vi "dummy RPM.vi"() -> ()   [LabVIEW 2018]
uses:
  <vilib>/DAQmx/write.llb/DAQmx Write (Counter Frequency 1Chan 1Samp).vi
  <vilib>/addons/control/pid/NI_PID_pid.lvlib
  <vilib>/DAQmx/configure/timing.llb/DAQmx Timing (Implicit).vi
  <vilib>/addons/control/pid/_prctrl compat.llb/PID (Compatibility).vi
  <vilib>/addons/control/pid/NI_PID__prctrl compat.lvlib
  <vilib>/DAQmx/read.llb/DAQmx Read (Counter DBL 1Chan 1Samp).vi
  <vilib>/addons/control/pid/pid.llb/PID Percentage to EGU (DBL).vi
panel:
  out "error":dbl
  in  "PID parameters":cluster{"Kp":dbl, "Ti":dbl, "Td":dbl}={"Kp"=1.0, "Ti"=0.0, "Td"=0.0} {"Td" format="%.2f"; "Ti" format="%.2f"; "Kp" format="%.2f"}
  out "Process Variable":dbl(knob) scale=0.0..180.0
  in  "Setpoint":dbl(knob) scale=0.0..180.0
  in  "frequency":dbl=1.0 format="%_6g"
  out "Respuesta":cluster{"Setpoint":dbl, "RPM":dbl, dbl}(graph)
  in  "stop":bool
  # "Proportional gain or band (Kc)"
  # "Integral (reset) time (Ti, min)"
  # "Derivative (rate) time (Td, min)"
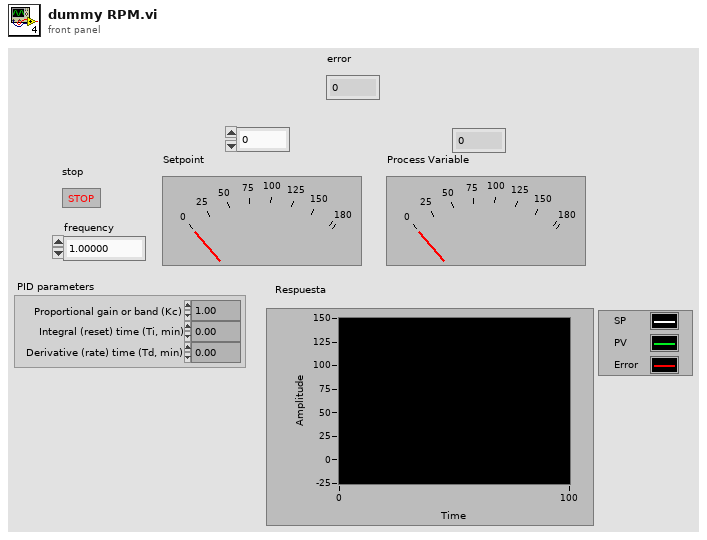
[diagram p1: front panel]
types:
  T1 = cluster{"sp low":dbl, "sp high":dbl, "out low":dbl, "out high":dbl, "hold (F)":bool, "auto (T)":bool, "pro. band (F)":bool, "reverse acting (T)":bool, "beta":dbl, "linearity":dbl, "dt (s)":dbl}
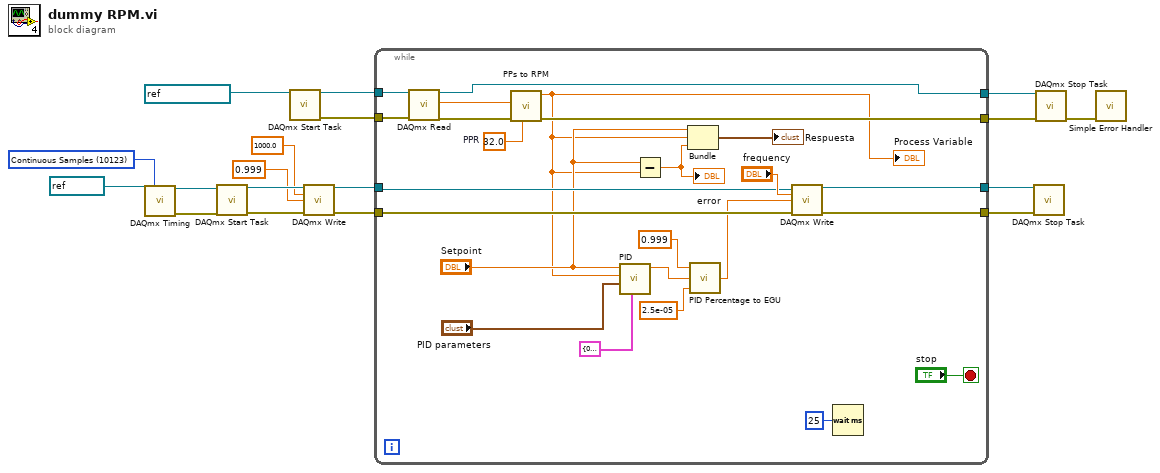
[diagram p0: block diagram]
diagram:
  w12 = 10123 items=["Finite Samples"=10178, "Continuous Samples"=10123, "Hardware Timed Single Point"=12522] ("sample mode")
  n1 = call-poly <vilib>:"DAQmx Timing.vi"("task/channels in"=refnum<k21> "CCW" ("DAQmx Global Channel"), "sample mode"=w12) -> ("task out"=w10:refnum<k21>, "error out"=w9:errorcluster)  [unwired: 12 in]
  n2 = call <vilib>:"DAQmx Start Task.vi"("task/channels in"=w10, "error in"=w9) -> ("task out"=w8:refnum<k21>, "error out"=w7:errorcluster)  [unwired: 12 in]
  n3 = call <vilib>:"DAQmx Start Task.vi"("task/channels in"=refnum<k21> "Tacometro" ("DAQmx Task Name")) -> ("task out"=w17:refnum<k21>, "error out"=w14:errorcluster)  [unwired: 13 in]
  n4 = call-poly <vilib>:"DAQmx Write.vi"("task/channels in"=w8, "frequency"=1000.0, "duty cycle"=0.999, "error in"=w7) -> ("task out"=w5:refnum<k21>, "error out"=w6:errorcluster)  [unwired: 9 in, 1 out]
  n5 = while {
    tunnel: w17 -> [w41]
    tunnel: [w40] -> w16
    tunnel: w14 -> [w39]
    tunnel: [w36] -> w13
    tunnel: w6 -> [w29]
    tunnel: w5 -> [w32]
    tunnel: [w28] -> w2
    tunnel: [w27] -> w1
    stop <- "stop" stop-if-true
    w35 = 32.0  # PPR
    n6 = call-poly <vilib>:"DAQmx Read.vi"("task/channels in"=w41, "error in"=w39) -> ("task out"=w40:refnum<k21>, "data"=w34:dbl, "error out"=w37:errorcluster)  [unwired: 11 in]
    n7 = call "PPs to RPM.vi"("PPR"=w35, "error in (no error)"=w37, "Speed (Hz)"=w34) -> ("error out"=w36:errorcluster, "RPM"=w21:dbl)  [unwired: 7 in]
    "Process Variable" <- w21
    n8 = call-poly <vilib>:"PID.vi"("options"=T1 {"sp low"=0.0, "sp high"=180.0, "out low"=0.0, "out high"=100.0, "hold (F)"=FALSE, "auto (T)"=TRUE, "pro. band (F)"=FALSE, "reverse acting (T)"=TRUE, "beta"=1.0, "linearity"=1.0, "dt (s)"=-1.0}, "PID parameters"="PID parameters", "process variable"=w21, "setpoint"="Setpoint") -> ("output"=w26:dbl)  [unwired: 7 in]
    n9 = Subtract(x="Setpoint", y=w21) -> (x-y=w20:dbl)
    "error" <- w20
    n10 = Bundle("Setpoint"="Setpoint", "RPM"=w21, w20) -> (→"Respuesta":cluster{"Setpoint":dbl, "RPM":dbl, dbl})  [unwired: 1 in]
    n11 = call-poly <vilib>:"PID Percentage to EGU.vi"("minimum (EGU)"=2.5e-05, "% span"=w26, "maximum (EGU)"=0.999) -> ("output (EGU)"=w23:dbl)  [unwired: 1 in]
    n12 = call-poly <vilib>:"DAQmx Write.vi"("task/channels in"=w32, "frequency"="frequency", "duty cycle"=w23, "error in"=w29) -> ("task out"=w27:refnum<k21>, "error out"=w28:errorcluster)  [unwired: 9 in, 1 out]
    n13 = Wait (ms)(milliseconds to wait=u32 25) -> ()  [unwired: 1 out]
  }
  n14 = call <vilib>:"DAQmx Stop Task.vi"("task/channels in"=w1, "error in"=w2) -> ()  [unwired: 12 in, 2 out]
  n15 = call <vilib>:"DAQmx Stop Task.vi"("task/channels in"=w16, "error in"=w13) -> ("error out"=w15:errorcluster)  [unwired: 12 in, 1 out]
  n16 = call <vilib>:"Simple Error Handler.vi"("error in (no error)"=w15) -> ()  [unwired: 4 in, 5 out]
